vi "Generate Event.vi"(8 "error in (no error)":errorcluster, 10 "TAS Event Data In":refnum<class "TAS_Event.lvclass">, 11 "TAS Event Refnum In":refnum<user-event>) -> (0 "error out":errorcluster, 3 "TAS Event Refnum Out":refnum<user-event>)   [LabVIEW 2012, in "TAS_Event.lvclass"]
uses:
  TAS_Event.lvclass
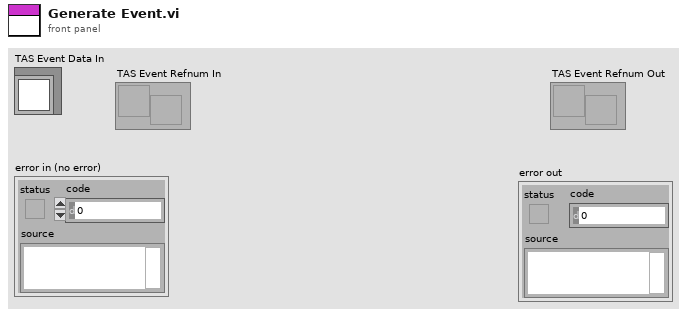
[diagram p1: front panel]
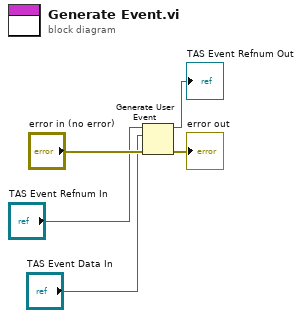
[diagram p0: block diagram]
diagram:
  n1 = Generate User Event(user event="TAS Event Refnum In", event data cluster="TAS Event Data In", error in="error in (no error)") -> (user event out=→"TAS Event Refnum Out":refnum<user-event>, error out=→"error out":errorcluster)
